vi "Read Float Parameter.vi"(8 "error in (no error)":errorcluster, 10 "Parameter Name":string, 11 "VoiceMeeterRemote in":refnum<class "VoiceMeeterRemote.lvclass">) -> (0 "error out":errorcluster, 2 "Value":sgl, 3 "VoiceMeeterRemote out":refnum<class "VoiceMeeterRemote.lvclass">)   [LabVIEW 2020, in "VoiceMeeterRemote.lvlib" / "VoiceMeeterRemote.lvclass"]
doc: "Reads a float parameter by name. See the VoiceMeeterRemote API manual for available parameters."
uses:
  VoiceMeeterRemote.lvclass
  VoiceMeeterRemote.lvclass/VoiceMeeterRemote.ctl
  VoiceMeeterRemote.lvlib
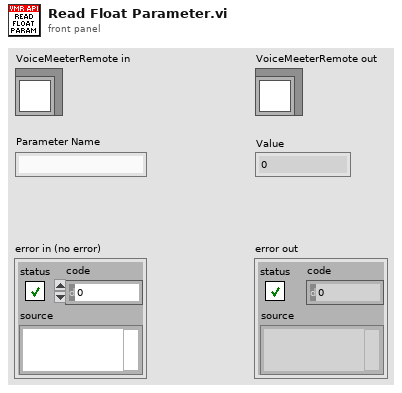
[diagram p1: front panel]
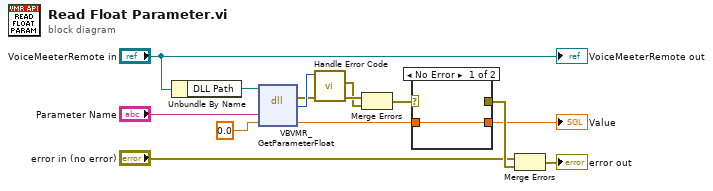
[diagram p0: block diagram]
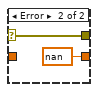
[diagram p2: hidden frame]
diagram:
  n1 = Unbundle By Name("VoiceMeeterRemote in") -> ("DLL Path"=w10:path)
  n2 = dll-call lib="C:/Program Files/National Instruments/LabVIEW 2022/user.lib/VoicemeeterRemote64/VoicemeeterRemote64.*" fn="VBVMR_GetParameterFloat"(path in=w10, "szParamName"="Parameter Name", "pValue"=sgl 0.0) -> (error out=w7:errorcluster, "return type"=w8:i32, "pValue"=w3:sgl)  [unwired: 3 in, 1 out]
  n3 = call "Handle Error Code.vi"("Code"=w8) -> ("error out"=w6:errorcluster)  [unwired: 10 in]
  n4 = Merge Errors(w7, w6) -> (w4:errorcluster)
  n5 = case shown="No Error" w4 {
    selector: w4 -> [_ w16]
    tunnel: w3 -> [w14 _]
    tunnel: [w14 sgl nan ("pValue")] -> w2
    tunnel: [_ w16] -> w13
    frame No Error {
    }
    frame Error {
    }
  }
  "Value" <- w2
  n6 = Merge Errors("error in (no error)", w13) -> (→"error out":errorcluster)
  "VoiceMeeterRemote out" <- "VoiceMeeterRemote in"
